vi "Autotune_Controlador_PID_bak1.vi"() -> ()   [LabVIEW 2013]
uses:
  <vilib>/addons/control/pid/autopid.llb/PID autotuning parameters.ctl
  <vilib>/Simulation/Scripting/Companion Diagram/SimConfigNode/SimParams.ctl
  <vilib>/Simulation/Scripting/Companion Diagram/SimConfigNode/_simSolvers.ctl
  <vilib>/Simulation/Implementation/Shared/SIMSCR Execution Mode.ctl
  <vilib>/Simulation/Param Hierarchy/Typedefs/SIMPH Param Control Actions.ctl
  <vilib>/Simulation/Implementation/Shared/NILVSim_ParamChanged.vi
  <vilib>/Simulation/Implementation/Shared/NILVSIM_BeginStep.vi
  <vilib>/Simulation/SignalArithmetic/Implementation/NILVSim Gain.llb/SIM Gain (scalar).vi
  <vilib>/Simulation/SignalDisplay/Implementation/NILVSim Time Waveform.llb/SIM Time Waveform (scalar).vi
  <vilib>/Simulation/Implementation/Shared/NILVSim_Manager.vi
  <vilib>/Simulation/Implementation/Shared/NILVSim_FinalizeModel.vi
  <vilib>/Simulation/Implementation/Shared/SIM Unbundle Sim Info.vi
  <vilib>/Utility/error.llb/Clear Errors.vi
  <vilib>/Simulation/Implementation/Shared/NILVSim_GetModelError.vi
  <vilib>/Simulation/Implementation/Shared/SIM Bundle Sim Info.vi
  <vilib>/Simulation/Implementation/Shared/SIMSH Read Queue.vi
  <vilib>/Simulation/Implementation/Shared/NILVSim_Initialize.vi
  <vilib>/Simulation/Utility/Implementation/NILVSim Get Time and IsAcceptedStep.vi
  <vilib>/addons/control/pid/autopid.llb/PID Online Autotuning.vi
  <vilib>/addons/control/pid/autopid.llb/PID Online Autotuning (PID on the loop).VI
  <vilib>/addons/control/pid/pid.llb/PID.vi
  <vilib>/addons/control/pid/pid.llb/PID (DBL).vi
  <vilib>/Simulation/Scripting/Companion Diagram/SimConfigNode/SimDog.xnode
  <vilib>/Simulation/Implementation/XNodeFramework/SimXNode/SimX.xnode
  <vilib>/addons/control/pid/NI_PID_pid.lvlib
  <vilib>/addons/control/pid/NI_PID_autopid.lvlib
  <vilib>/Simulation/Implementation/Shared/NI_SIM_Implementation.lvlib
panel:
  out "Boolean 2":bool
  in  "Boolean":bool
  out "tuned PID gains":T1={"proportional gain (Kc)"=1.0, "integral time (Ti, min)"=0.01, "derivative time (Td, min)"=0.0} {"derivative time (Td, min)" format="%.3f"; "integral time (Ti, min)" format="%.3f"; "proportional gain (Kc)" format="%.3f"}
  in  "autotuning parameters":T2={"type of controller"=1, "relay cycles"=3, "relay amplitude"=1.0, "control specifications"=2, "PV noise level"=0.1} {"PV noise level" format="%.2f"; "control specifications" items=["Fast", "Normal", "Slow"]; "relay amplitude" format="%.2f"; "type of controller" items=["P", "PI", "PID"]}
  in  "runned":bool
  in  "restart":bool
  in  "stop":bool
  out "Sinal de controle [%]":waveform(dbl)(graph)
  out "Waveform INPUT":dynamicdata(graph)=[{"t0"=timestamp(3771854592.7277975 s since 1904-01-01), "dt"=1.0, "Y"=[-4.527297247023809], "attributes"=variant("NI_ChannelName"=variant(string "Filtered"))}]
  in  "SV":dbl=50.0
  out "PID gains out":T1={"proportional gain (Kc)"=1.0, "integral time (Ti, min)"=0.01, "derivative time (Td, min)"=0.0} {"derivative time (Td, min)" format="%.3f"; "integral time (Ti, min)" format="%.3f"; "proportional gain (Kc)" format="%.3f"}
  out "tuning completed?":bool
  in  "AUTOTUNE":bool
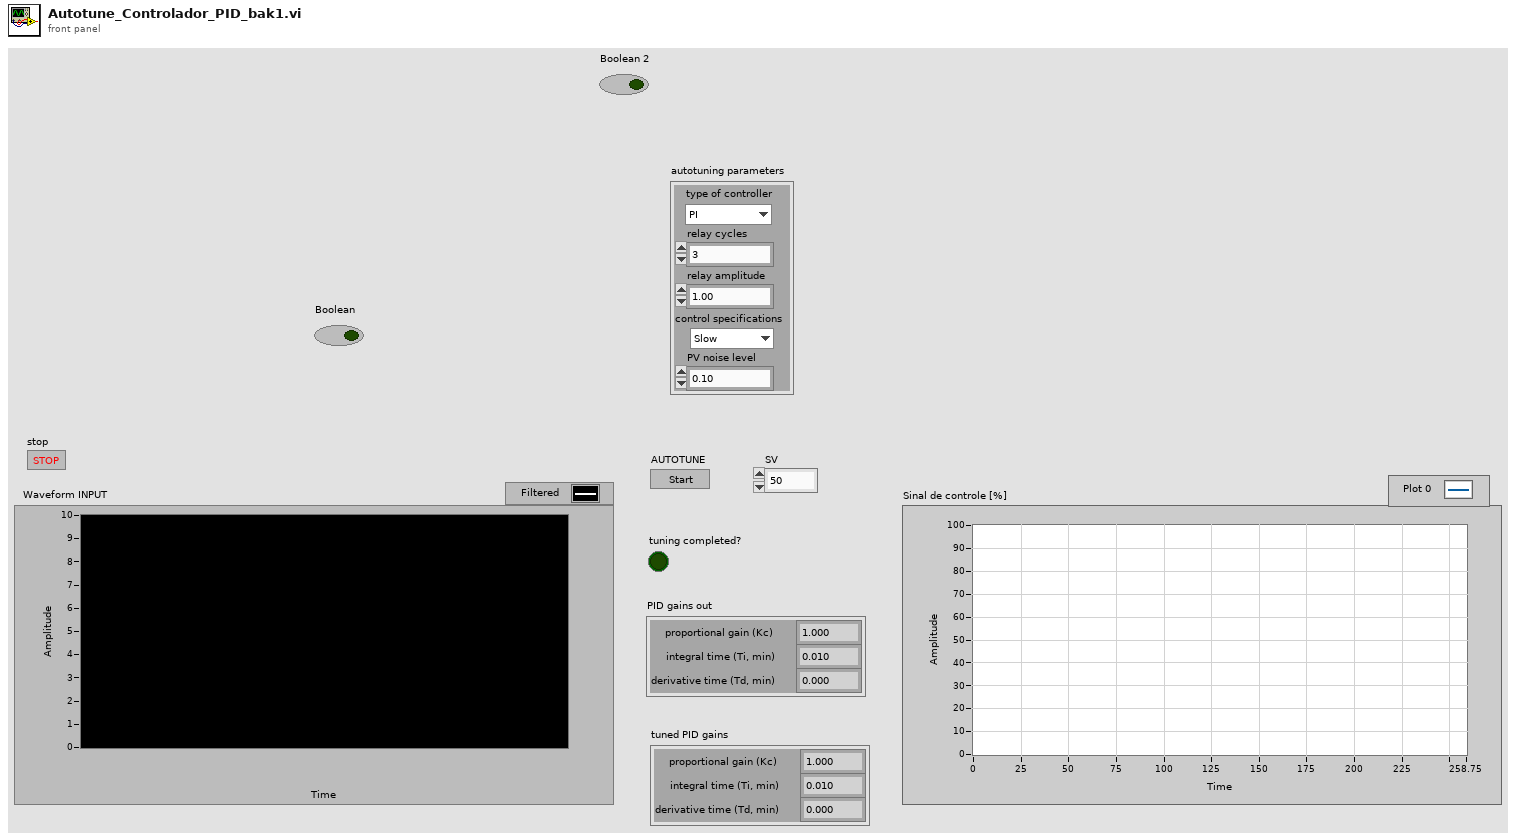
[diagram p1: front panel]
types:
  T1 = cluster{"proportional gain (Kc)":dbl, "integral time (Ti, min)":dbl, "derivative time (Td, min)":dbl}
  T2 = typedef "PID autotuning parameters.ctl" = cluster{"type of controller":u16, "relay cycles":i32, "relay amplitude":dbl, "control specifications":u16, "PV noise level":dbl}
  T3 = typedef "SIMSCR Execution Mode.ctl" = enum16{"Simulate to Completion", "Single Time-Step Simulation (Fixed Step Only)"}
  T4 = typedef "SIMPH Param Control Actions.ctl" = enum16{"get params", "set params"}
  T5 = typedef "SimParams.ctl" = cluster{"Initial Time (s)":dbl, "Final Time (s)":dbl, "Step Size (s)":dbl, "ODE Solver":T6, "Minimum Step Size (s)":dbl, "Maximum Step Size (s)":dbl, "Relative Tolerance":dbl, "Absolute Tolerance":dbl, "Software Timing":bool, "Initial Step Size (s)":dbl, "Automatic Fixed Step Size?":bool, "Automatic Discrete Step Size?":bool, "Discrete Step Size (s)":dbl, "Calculate using Time Step":bool, "Solver Wired?":bool, "Prev.Frm.Expected End":u64, "Prev.Frm.Actual End":u64, "Prev.Frm.Finished Late?":bool, "Prev.Iter.Expected End":u64, "Prev.Iter.Actual End":u64, "Prev.Iter.Finished Late?":bool, "Expected Iteration Start":u64, "Actual Iteration Start":u64, "Expected Frame Start":u64, "Actual Frame Start":u64, "Source Name":string, "Name":string, "Period":i64, "Deadline":i64, "Offset":i64, "Start":i64, "Priority":i32, "Timeout":i32, "Processor":i32, "Mode":enum32{"No Change", "Process missed periods, maintain original phase", "Discard missed periods, maintain original phase", "Process missed periods, ignore original phase", "Discard missed periods, ignore original phase"}, "Wakeup reason":enum32{"Normal", "Aborted", "Asynchronous wakeup", "Timing source error", "Timed loop error", "Timeout"}, "Error":errorcluster, "Source Type":string, "Secondary Source Type":string, "Global End Time":u64, "Global Start Time":u64, "Full Solver Reset":bool, "Execution Mode":T3, "Nan/Inf Check":bool, "Custom Solver Library":string, "Solver Is Variable":bool, "custom solver name":string, "Signal Collection Decimation":u32}
  T6 = typedef "_simSolvers.ctl" = enum16{"Runge-Kutta 1 (Euler)", "Runge-Kutta 2", "Runge-Kutta 3", "Runge-Kutta 4", "Runge-Kutta 23 (variable)", "Runge-Kutta 45 (variable)", "BDF (variable)", "Adams-Moulton (variable)", "Rosenbrock (variable)", "Discrete States Only", "SDIRK 4 (variable)", "Radau 5 (variable)", "Radau 9 (variable)", "Radau 13 (variable)", "Radau [Variable Order] (variable)", "Gear's Method (variable)", "Linearizer", "State Query", "Trim Eval", "Custom Solver"}
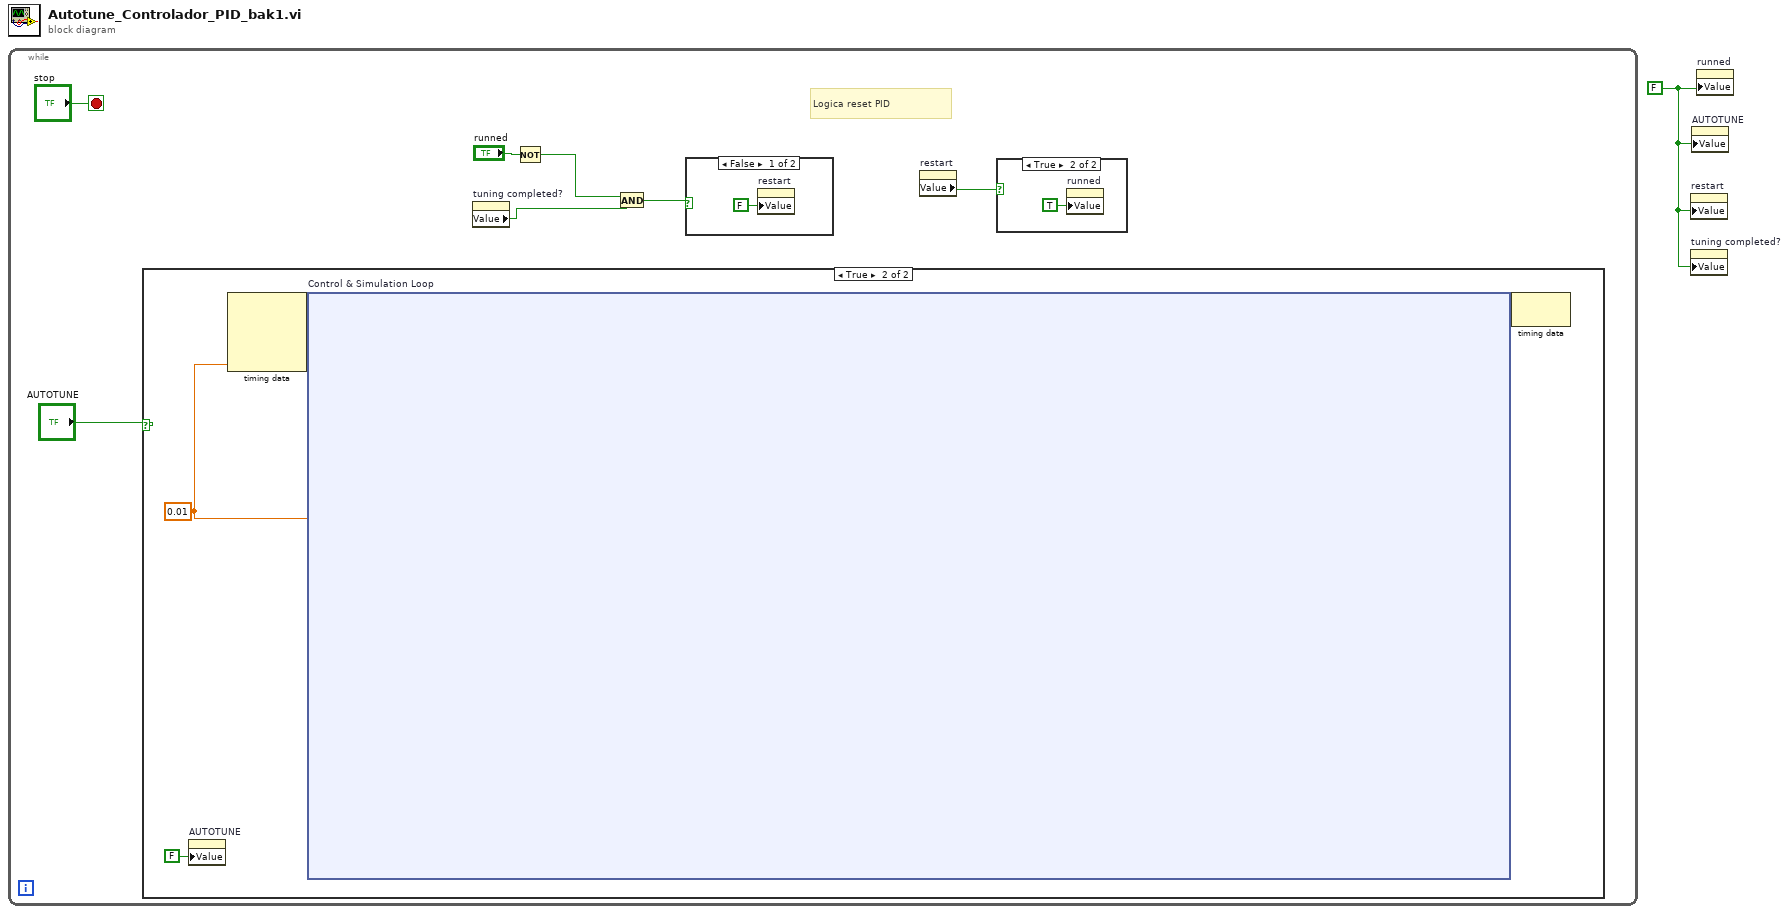
[diagram p0: block diagram]
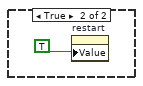
[diagram p3: hidden frame]
diagram:
  w1 = FALSE ("Simulate")
  n1 = while {
    stop <- "stop" stop-if-true
    # "Logica reset PID"
    n2 = case shown="True" "AUTOTUNE" {
      frame False {
      }
      frame True {
        w12 = 0.01 ("Step Size (s)")
        n3 = property on="AUTOTUNE" class="Bool (strict)"("Value"=FALSE ("Simulate")) -> ()  [unwired: 2 in, 2 out]
        n4 = node-c288(w12) -> (w15:variant)  [unwired: 3 in]
        n5 = node-c254 "Control & Simulation Loop"(w15, w12) -> (w14:variant)
        n6 = node-c288(w14) -> ()  [unwired: 1 out]
      }
    }
    n7 = property on="tuning completed?" class="Bool (strict)"() -> ("Value"=w2:bool)  [unwired: 2 in, 2 out]
    n8 = Not(x="runned") -> (.not. x?=w4:bool)
    n9 = And(x=w4, y=w2) -> (x .and. y?=w6:bool)
    n10 = case shown="False" w6 {
      frame False {
        n11 = property on="restart" class="Bool (strict)"("Value"=FALSE ("restart 5")) -> ()  [unwired: 2 in, 2 out]
      }
      frame True {
        n12 = property on="restart" class="Bool (strict)"("Value"=TRUE ("restart 6")) -> ()  [unwired: 2 in, 2 out]
      }
    }
    n13 = property on="restart" class="Bool (strict)"() -> ("Value"=w3:bool)  [unwired: 2 in, 2 out]
    n14 = case "Case Structure 2" shown="True" w3 {
      frame False {
      }
      frame True {
        n15 = property on="runned" class="Bool (strict)"("Value"=TRUE ("first")) -> ()  [unwired: 2 in, 2 out]
      }
    }
  }
  n16 = property on="restart" class="Bool (strict)"("Value"=w1) -> ()  [unwired: 2 in, 2 out]
  n17 = property on="tuning completed?" class="Bool (strict)"("Value"=w1) -> ()  [unwired: 2 in, 2 out]
  n18 = property on="AUTOTUNE" class="Bool (strict)"("Value"=w1) -> ()  [unwired: 2 in, 2 out]
  n19 = property on="runned" class="Bool (strict)"("Value"=w1) -> ()  [unwired: 2 in, 2 out]
